vi "Live window-Tick boxes visibility state.vi"(8 "error in (no error)":errorcluster) -> (0 "error out":errorcluster)   [LabVIEW 2017]
uses:
  Typedefs/HW config states enum.ctl
  Global Variables/General Globals.vi
  Globals/gl_Windows Ctrl refs.vi
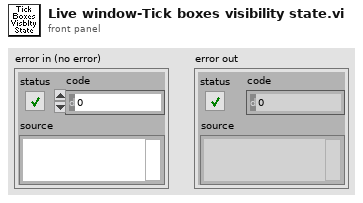
[diagram p1: front panel]
types:
  T1 = typedef "HW config states enum.ctl" = enum16{"Load from file", "Save to file", "Write all", "Read all", "Write XY stage settings", "Write DAQ FPGA settings", "Write Control FPGA settings", "Write Phys Channels", "Clear", "Compare from file"}
  T2 = typedef "Hardware Configuration settings.ctl" = cluster{"Computer MAC address":string, "XY Stage":T3, "Cam VidRec":T4, "Control Sys. HW config":T5, "DAQ FPGA HW Config":cluster{"Target":T6, "input card type":T7}, "DAQmx Chan":T8, "Encoder":T9, "Z Stage config cluster":T10, "Trigger HW config":T11, "Externalise Triggers":bool, "MC Supported":bool, "Laser 1 config cluster":T12, "Prechirper 1 config cluster":T13, "Laser Power Control HW config":T14, "No of AOD":u8, "Dev. PC":bool, "Swap XY on stage":bool, "Axial MC":bool}
  T3 = typedef "XY Stage config cluster.ctl" = cluster{"COM port":refnum<visa-resource-name>, "XY stage available":bool, "Baudrate":i32, "Type":string}
  T4 = typedef "Cam VidRec HW config setup cluster.ctl" = cluster{"DO flag-Video record":tag, "DO flag-Trial start":tag, "VidRec available":bool}
  T5 = typedef "Control Sys HW config cluster.ctl" = cluster{"Control system.FPGA available?":bool, "Control system.FPGA Type":string, "Control system.Network adapter name":string, "Control system.MAC address":string, "Control system.Ethernet Port":u32}
  T6 = typedef "nirio_resource_hc.ctl" = tag
  T7 = typedef "FPGA input type AC-DC.ctl" = enum16{"AC Card", "DC Card"}
  T8 = typedef "DAQmx physical channels cluster.ctl" = cluster{"Pockels AO":tag, "Hard shutter AO":tag, "PMT AOs":tag, "Power meter AI":tag}
  T9 = typedef "Encoder config cluster.ctl" = cluster{"IP address":string, "Port":u16, "Encoder available":bool, "Wheel radius (cm)":dbl, "Encoder Trigger":tag}
  T10 = typedef "Z Stage config cluster.ctl" = cluster{"COM port":refnum<visa-resource-name>, "Z stage available":bool, "Baudrate":i32, "Type":string}
  T11 = typedef "Triggers HW config.ctl" = cluster{"Available Device List":i32, "Device Address":string}
  T12 = typedef "Laser 1 config cluster.ctl" = cluster{"COM port":refnum<visa-resource-name>, "Laser 1 available":bool, "Baud Rate":i32, "Type":string}
  T13 = typedef "PreChirper 1 config cluster.ctl" = cluster{"COM port":refnum<visa-resource-name>, "Prechirper 1 \navailable":bool, "Baud Rate":i32, "Type":string}
  T14 = typedef "Laser Power Control HW config.ctl" = cluster{"Laser Power Control":string, "Laser Power Modulation Control":string}
  T15 = typedef "Live window-ctrl refs.ctl" = cluster{"This VI":refnum<vi>, "Pane":refnum<vi>, "Show REF Image Left":refnum<vi>, "Show REF Image Right":refnum<vi>, "Snapshot":refnum<vi>, "Left Image Palette":refnum<vi>, "Right Image Palette":refnum<vi>, "Left Channel":refnum<vi>, "Right Channel":refnum<vi>, "Left image intensity":refnum<vi>, "Right image intensity":refnum<vi>, "Left Image Display":T16, "Right Image Display":T16, "Refresh rate ind (Hz)":refnum<vi>, "Acq rate ind (Hz)":refnum<vi>, "Stop (ind)":refnum<vi>}
  T16 = typedef "Image display ref.ctl" = refnum<vi>
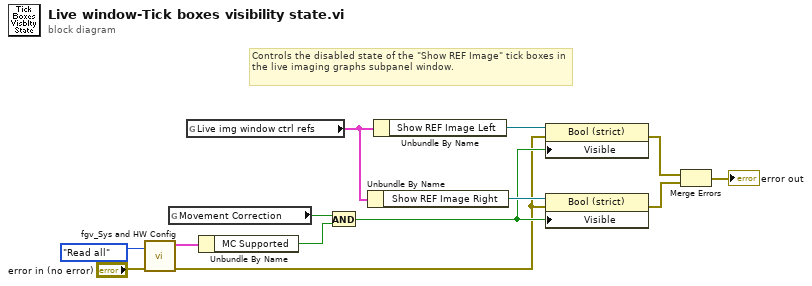
[diagram p0: block diagram]
diagram:
  # "Controls the disabled state of the \"Show REF Image\" tick boxes in the live imaging graphs subpanel window."
  n1 = call "fgv_Sys and HW Config.vi"("Function"=HW_config_states_enum."Read all", "error in (no error)"="error in (no error)") -> ("error out"=w4:errorcluster, "Hardware Configuration OUT"=w10:T2)  [unwired: 7 in, 1 out]
  n2 = global read "General Globals.vi" "Movement Correction"() -> (w7:bool)
  n3 = global read "gl_Windows Ctrl refs.vi" "Live img window ctrl refs"() -> (w6:T15)
  n4 = Unbundle By Name(w10) -> ("MC Supported"=w8:bool)
  n5 = And(x=w7, y=w8) -> (x .and. y?=w11:bool)
  n6 = Unbundle By Name(w6) -> ("Show REF Image Right"=w12:refnum<vi>)
  n7 = Unbundle By Name(w6) -> ("Show REF Image Left"=w13:refnum<vi>)
  n8 = property on="Property Node" class="Bool (strict)"(reference=w13, error in=w4, "Visible"=w11) -> (error out=w3:errorcluster)  [unwired: 1 out]
  n9 = property on="Property Node" class="Bool (strict)"(reference=w12, error in=w4, "Visible"=w11) -> (error out=w2:errorcluster)  [unwired: 1 out]
  n10 = Merge Errors(w3, w2) -> (→"error out":errorcluster)
